vi "Get Model Info - from SysDef.vi"(0 "System Definition Filepath (.nivssdf)":path, 1 "Model Ref":refnum<k24>, 5 "Error (in)":errorcluster, 6 "Append Full Path?":bool) -> (13 "Model Path":path, 14 "SysDef Inports":string[](array[string]), 15 "SysDef Outports":string[](array[string]), 16 "SysDef Parameters":string[](array[string]), 17 "SysDef Signals":string[](array[string]), 18 "Model Name":string, 19 "Error (out)":errorcluster)   [LabVIEW 2016, in "System Mapping Tool.lvlib"]
uses:
  System Mapping Tool.lvlib
  NationalInstruments.VeriStand.SystemDefinitionAPI
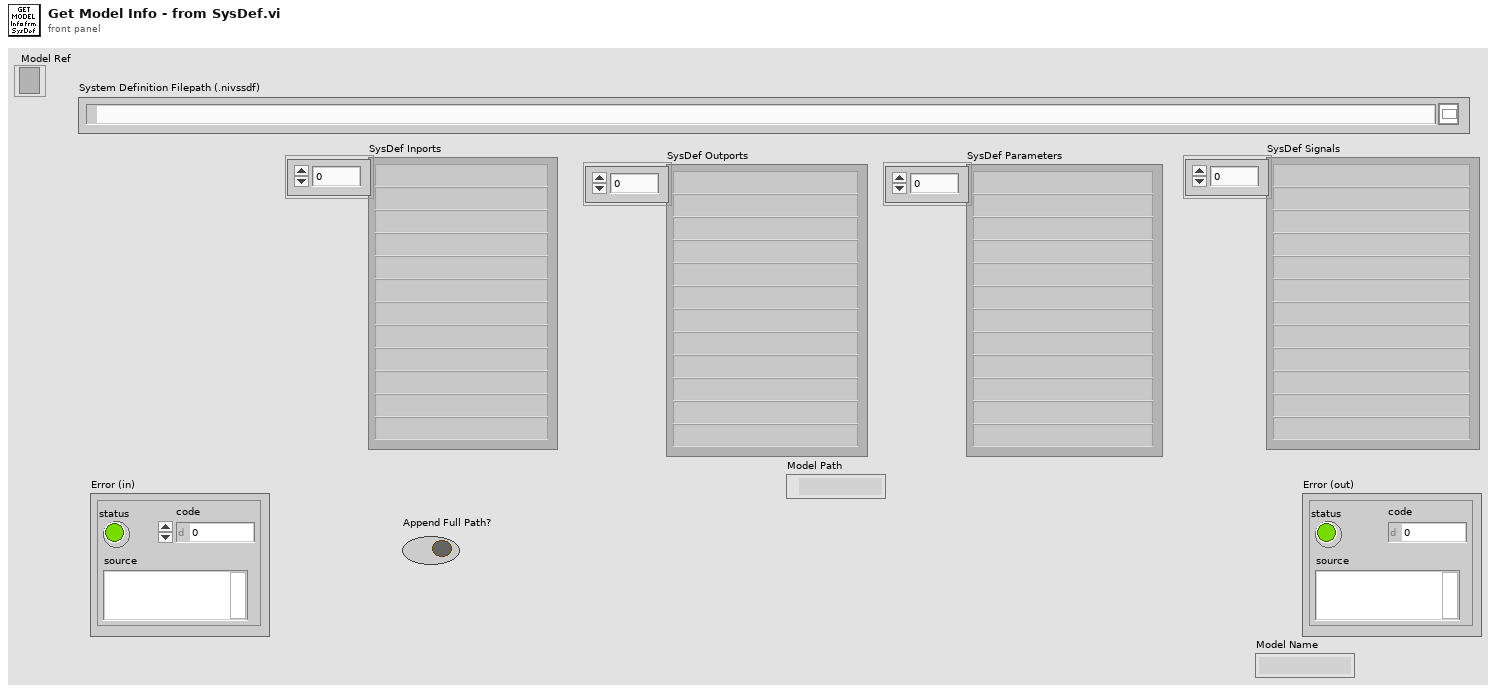
[diagram p1: front panel]
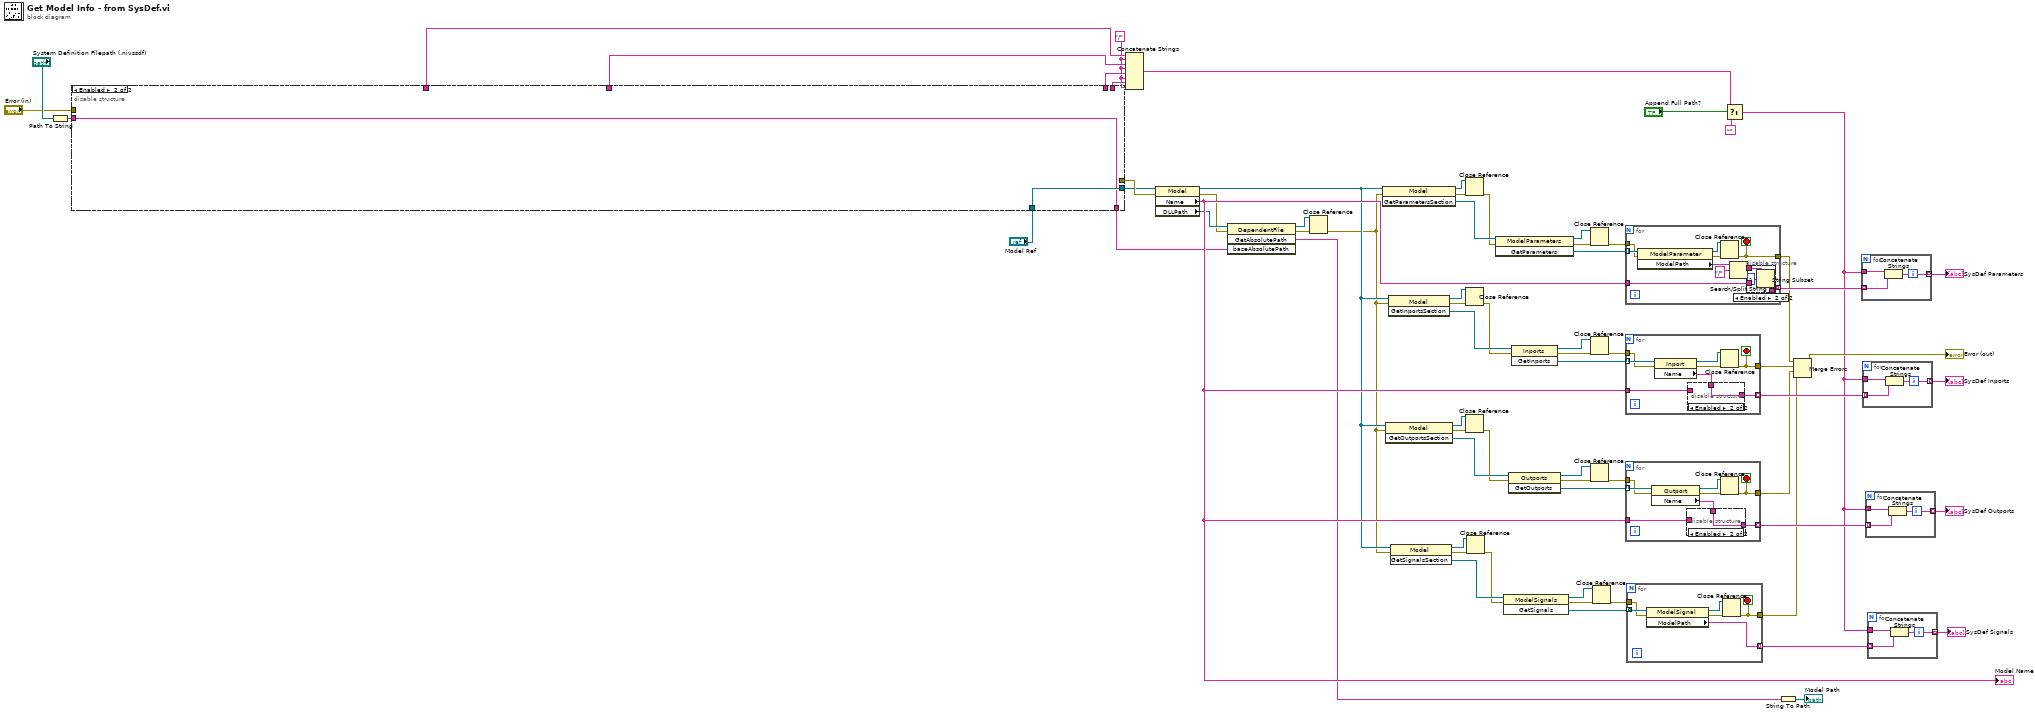
[diagram p0: block diagram]
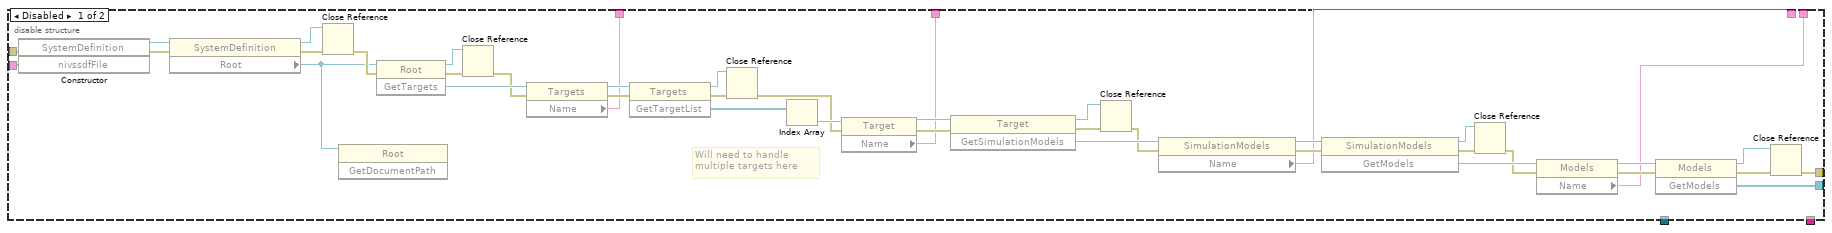
[diagram p2: hidden frame]
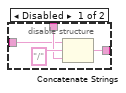
[diagram p3: hidden frame]
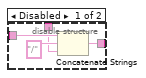
[diagram p4: hidden frame]
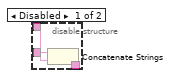
[diagram p5: hidden frame]
diagram:
  w60 = "/"
  n1 = Path To String(path="System Definition Filepath (.nivssdf)") -> (string=w69:string)
  n2 = disable-structure shown="Enabled" {
    disable-tunnel: w69 -> [w111 w112]
    disable-tunnel: [w108 w113] -> w4
    disable-tunnel: [w95 _] -> w68
    disable-tunnel: "Error (in)" -> [w93 _]
    disable-tunnel: [w75 _] -> w64
    disable-tunnel: [w74 _] -> w63
    disable-tunnel: [w73 _] -> w62
    disable-tunnel: [w72 _] -> w61
    disable-tunnel: "Model Ref" -> [_ w113]
    disable-tunnel: [_ w112] -> w1
    frame Disabled {
      # "Will need to handle multiple targets here"
      n3 = constructor class="SystemDefinition"(error in=w93, "nivssdfFile"=w111) -> (reference out=w110:refnum<k24>, error out=w109:errorcluster)  [unwired: 2 in, 2 out]
      n4 = property class="SystemDefinition"(reference=w110, error in=w109) -> (reference out=w106:refnum<k24>, error out=w105:errorcluster, "Root"=w71:refnum<k24>)
      n5 = Close Reference(reference=w106, error in (no error)=w105) -> (error out=w104:errorcluster)
      n6 = invoke class="Root" method="GetDocumentPath"(reference=w71) -> ()  [unwired: 2 in, 3 out]
      n7 = invoke class="Root" method="GetTargets"(reference=w71, error in=w104) -> (reference out=w102:refnum<k24>, error out=w89:errorcluster, "GetTargets"=w92:refnum<k24>)  [unwired: 1 in]
      n8 = Close Reference(reference=w102, error in (no error)=w89) -> (error out=w88:errorcluster)
      n9 = property class="Targets"(reference=w92, error in=w88) -> (reference out=w90:refnum<k24>, error out=w87:errorcluster, "Name"=w75:string)
      n10 = invoke class="Targets" method="GetTargetList"(reference=w90, error in=w87) -> (reference out=w101:refnum<k24>, error out=w103:errorcluster, "GetTargetList"=w107:refnum<k24>[])  [unwired: 1 in]
      n11 = Close Reference(reference=w101, error in (no error)=w103) -> (error out=w85:errorcluster)
      n12 = Index Array(array=w107) -> (element=w86:refnum<k24>)  [unwired: 1 in]
      n13 = property class="Target"(reference=w86, error in=w85) -> (reference out=w84:refnum<k24>, error out=w83:errorcluster, "Name"=w74:string)
      n14 = invoke class="Target" method="GetSimulationModels"(reference=w84, error in=w83) -> (reference out=w99:refnum<k24>, error out=w100:errorcluster, "GetSimulationModels"=w91:refnum<k24>)  [unwired: 1 in]
      n15 = Close Reference(reference=w99, error in (no error)=w100) -> (error out=w82:errorcluster)
      n16 = property class="SimulationModels"(reference=w91, error in=w82) -> (reference out=w81:refnum<k24>, error out=w80:errorcluster, "Name"=w73:string)
      n17 = invoke class="SimulationModels" method="GetModels"(reference=w81, error in=w80) -> (reference out=w97:refnum<k24>, error out=w98:errorcluster, "GetModels"=w79:refnum<k24>)  [unwired: 1 in]
      n18 = Close Reference(reference=w97, error in (no error)=w98) -> (error out=w77:errorcluster)
      n19 = property class="Models"(reference=w79, error in=w77) -> (reference out=w78:refnum<k24>, error out=w76:errorcluster, "Name"=w72:string)
      n20 = invoke class="Models" method="GetModels"(reference=w78, error in=w76) -> (reference out=w94:refnum<k24>, error out=w96:errorcluster, "GetModels"=w108:refnum<k24>[])  [unwired: 1 in]
      n21 = Close Reference(reference=w94, error in (no error)=w96) -> (error out=w95:errorcluster)
    }
    frame Enabled {
    }
  }
  n22 = Concatenate Strings(w64, w60, w63, w60, w62, w60, w61, w60) -> (w52:string)
  n23 = property class="Model"(reference=w4, error in=w68) -> (reference out=w7:refnum<k24>, error out=w19:errorcluster, "Name"=w67:string, "DLLPath"=w20:refnum<k24>)
  "Model Name" <- w67
  n24 = invoke class="DependentFile" method="GetAbsolutePath"(reference=w20, error in=w19, "baseAbsolutePath"=w1) -> (reference out=w17:refnum<k24>, error out=w18:errorcluster, "GetAbsolutePath"=w16:string)  [unwired: 1 in, 1 out]
  n25 = Close Reference(reference=w17, error in (no error)=w18) -> (error out=w6:errorcluster)
  n26 = invoke class="Model" method="GetParametersSection"(reference=w7, error in=w6) -> (reference out=w44:refnum<k24>, error out=w45:errorcluster, "GetParametersSection"=w47:refnum<k24>)  [unwired: 1 in]
  n27 = invoke class="Model" method="GetOutportsSection"(reference=w7, error in=w6) -> (reference out=w28:refnum<k24>, error out=w29:errorcluster, "GetOutportsSection"=w31:refnum<k24>)  [unwired: 1 in]
  n28 = invoke class="Model" method="GetInportsSection"(reference=w7, error in=w6) -> (reference out=w36:refnum<k24>, error out=w37:errorcluster, "GetInportsSection"=w39:refnum<k24>)  [unwired: 1 in]
  n29 = invoke class="Model" method="GetSignalsSection"(reference=w7, error in=w6) -> (reference out=w12:refnum<k24>, error out=w13:errorcluster, "GetSignalsSection"=w15:refnum<k24>)  [unwired: 1 in]
  n30 = Close Reference(reference=w44, error in (no error)=w45) -> (error out=w43:errorcluster)
  n31 = Close Reference(reference=w36, error in (no error)=w37) -> (error out=w35:errorcluster)
  n32 = Close Reference(reference=w28, error in (no error)=w29) -> (error out=w27:errorcluster)
  n33 = Close Reference(reference=w12, error in (no error)=w13) -> (error out=w11:errorcluster)
  n34 = invoke class="ModelParameters" method="GetParameters"(reference=w47, error in=w43) -> (reference out=w40:refnum<k24>, error out=w42:errorcluster, "GetParameters"=w46:refnum<k24>[])  [unwired: 1 in]
  n35 = invoke class="ModelSignals" method="GetSignals"(reference=w15, error in=w11) -> (reference out=w8:refnum<k24>, error out=w10:errorcluster, "GetSignals"=w14:refnum<k24>[])  [unwired: 1 in]
  n36 = invoke class="Outports" method="GetOutports"(reference=w31, error in=w27) -> (reference out=w24:refnum<k24>, error out=w26:errorcluster, "GetOutports"=w30:refnum<k24>[])  [unwired: 1 in]
  n37 = invoke class="Inports" method="GetInports"(reference=w39, error in=w35) -> (reference out=w32:refnum<k24>, error out=w34:errorcluster, "GetInports"=w38:refnum<k24>[])  [unwired: 1 in]
  n38 = Close Reference(reference=w40, error in (no error)=w42) -> (error out=w41:errorcluster)
  n39 = Close Reference(reference=w32, error in (no error)=w34) -> (error out=w33:errorcluster)
  n40 = Close Reference(reference=w24, error in (no error)=w26) -> (error out=w25:errorcluster)
  n41 = Close Reference(reference=w8, error in (no error)=w10) -> (error out=w9:errorcluster)
  n42 = for {
    tunnel: w46 -> [w123] mode=indexing
    tunnel: [w118] -> w58 mode=indexing
    tunnel: w41 -> [w122]
    tunnel: [w120] -> w23
    tunnel: w67 -> [w117]
    stop <- w120 stop-if-true
    n43 = property class="ModelParameter"(reference=w123, error in=w122) -> (reference out=w119:refnum<k24>, error out=w121:errorcluster, "ModelPath"=w115:string)
    n44 = Close Reference(reference=w119, error in (no error)=w121) -> (error out=w120:errorcluster)
    n45 = Search/Split String(string=w115, search string/char (-)="/") -> (match + rest of string=w114:string)  [unwired: 1 in, 2 out]
    n46 = disable-structure shown="Enabled" {
      disable-tunnel: [w126 w128] -> w118
      disable-tunnel: w117 -> [w125 _]
      disable-tunnel: w114 -> [w124 w129]
      frame Disabled {
        n47 = Concatenate Strings(w125, w124) -> (w126:string)
      }
      frame Enabled {
        n48 = String Subset(string=w129, offset (0)=1) -> (substring=w128:string)  [unwired: 1 in]
      }
    }
  }
  n49 = for {
    tunnel: w38 -> [w137] mode=indexing
    tunnel: [w130] -> w57 mode=indexing
    tunnel: w33 -> [w136]
    tunnel: [w134] -> w22
    tunnel: w67 -> [w132]
    stop <- w134 stop-if-true
    n50 = property class="Inport"(reference=w137, error in=w136) -> (reference out=w133:refnum<k24>, error out=w135:errorcluster, "Name"=w131:string)
    n51 = disable-structure shown="Enabled" {
      disable-tunnel: w132 -> [w140 _]
      disable-tunnel: w131 -> [w139 w142]
      disable-tunnel: [w138 w142] -> w130
      frame Disabled {
        n52 = Concatenate Strings(w140, "/" ("string"), w139) -> (w138:string)
      }
      frame Enabled {
      }
    }
    n53 = Close Reference(reference=w133, error in (no error)=w135) -> (error out=w134:errorcluster)
  }
  n54 = for {
    tunnel: w30 -> [w150] mode=indexing
    tunnel: [w144] -> w54 mode=indexing
    tunnel: w25 -> [w149]
    tunnel: [w147] -> w21
    tunnel: w67 -> [w143]
    stop <- w147 stop-if-true
    n55 = property class="Outport"(reference=w150, error in=w149) -> (reference out=w146:refnum<k24>, error out=w148:errorcluster, "Name"=w145:string)
    n56 = disable-structure shown="Enabled" {
      disable-tunnel: w145 -> [w153 w155]
      disable-tunnel: [w152 w155] -> w144
      disable-tunnel: w143 -> [w151 _]
      frame Disabled {
        n57 = Concatenate Strings(w151, "/" ("string"), w153) -> (w152:string)
      }
      frame Enabled {
      }
    }
    n58 = Close Reference(reference=w146, error in (no error)=w148) -> (error out=w147:errorcluster)
  }
  n59 = for {
    tunnel: w14 -> [w161] mode=indexing
    tunnel: w9 -> [w160]
    tunnel: [w158] -> w5
    tunnel: [w156] -> w49 mode=indexing
    stop <- w158 stop-if-true
    n60 = property class="ModelSignal"(reference=w161, error in=w160) -> (reference out=w157:refnum<k24>, error out=w159:errorcluster, "ModelPath"=w156:string)
    n61 = Close Reference(reference=w157, error in (no error)=w159) -> (error out=w158:errorcluster)
  }
  n62 = Select(t=w52, s="Append Full Path?", f="") -> (s? t:f=w48:string)
  n63 = String To Path(string=w16) -> (path=→"Model Path":path)
  n64 = Merge Errors(w23, w22, w21, w5) -> (→"Error (out)":errorcluster)
  n65 = for {
    tunnel: [w164] -> w59 mode=indexing
    tunnel: w48 -> [w163]
    tunnel: w58 -> [w162] mode=indexing
    n66 = Concatenate Strings(w163, w162) -> (w164:string)
  }
  "SysDef Parameters" <- w59
  n67 = for {
    tunnel: [w167] -> w56 mode=indexing
    tunnel: w48 -> [w166]
    tunnel: w57 -> [w165] mode=indexing
    n68 = Concatenate Strings(w166, w165) -> (w167:string)
  }
  "SysDef Inports" <- w56
  n69 = for {
    tunnel: [w170] -> w55 mode=indexing
    tunnel: w48 -> [w169]
    tunnel: w54 -> [w168] mode=indexing
    n70 = Concatenate Strings(w169, w168) -> (w170:string)
  }
  "SysDef Outports" <- w55
  n71 = for {
    tunnel: [w173] -> w50 mode=indexing
    tunnel: w48 -> [w172]
    tunnel: w49 -> [w171] mode=indexing
    n72 = Concatenate Strings(w172, w171) -> (w173:string)
  }
  "SysDef Signals" <- w50
